vi "Release Card.vi"(8 "error in (no error)":errorcluster caption="错误输入（无错误）", 11 "CardNumber":u16) -> (0 "error out":errorcluster caption="错误输出", 3 "function return":i16)   [LabVIEW 2017, in "Adlink IO.lvlib"]
doc: "I16 __stdcall Release_Card(U16 CardNumber);"
uses:
  Adlink IO.lvlib
  PCI-Dask.dll
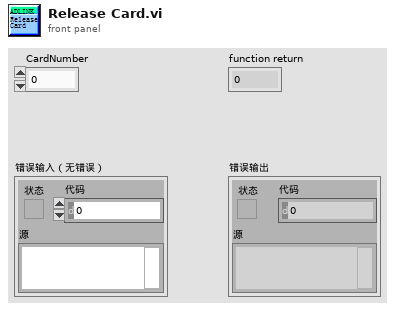
[diagram p1: front panel]
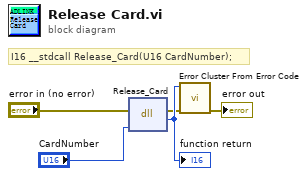
[diagram p0: block diagram]
diagram:
  # "I16 __stdcall Release_Card(U16 CardNumber);"
  n1 = dll-call lib="D:/Program/Dyson X692 UI Provison Tester V1.0.0/HardWare/ADLINK/IO/Adlink IO/PCI-Dask.*" fn="Release_Card"(error in="error in (no error)", "CardNumber"="CardNumber") -> (error out=w2:errorcluster, w5:i16)  [unwired: 3 in, 1 out]
  "function return" <- w5
  n2 = call <vilib>:"Error Cluster From Error Code.vi"("error in (no error)"=w2, "error code (0)"=w5) -> ("error out"=→"error out":errorcluster)  [unwired: 7 in]
